vi "celcius_to_farenheit.vi"() -> ()   [LabVIEW 2019]
panel:
  in  "celcius_slide":dbl(slide) scale=0.0..100.0
  in  "?":bool
  in  "celcius":dbl
  out "Farenheat":dbl
  # "CELSIUS TO FAREINHEAT"
  # "="
  # "(or)"
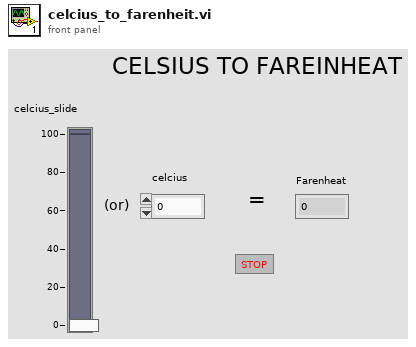
[diagram p1: front panel]
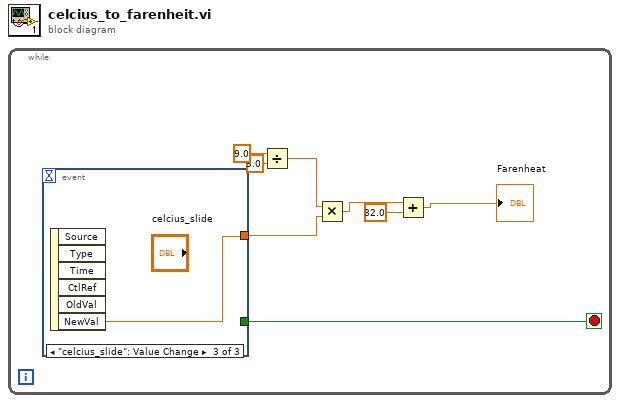
[diagram p0: block diagram]
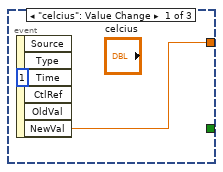
[diagram p2: hidden frame]
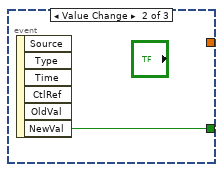
[diagram p3: hidden frame]
diagram:
  n1 = while {
    stop <- w1 stop-if-true
    n2 = event shown="[2] \"celcius_slide\": Value Change" {
      selector: _ -> [_ _ _]
      dyn-events: _ -> [_ _ _]
      timeout: _ -> [_ _ _]
      tunnel: [w9 _ w11] -> w2
      tunnel: [_ w10 _] -> w1
      event "celcius": Value Change {
        (unwired) u32 1 ("Time")
        n3 = event-data() -> ("NewVal"=w9:dbl)  [unwired: 1 in, 5 out]
      }
      event Value Change {
        n4 = event-data() -> ("NewVal"=w10:bool)  [unwired: 1 in, 5 out]
      }
      event "celcius_slide": Value Change {
        n5 = event-data() -> ("NewVal"=w11:dbl)  [unwired: 1 in, 5 out]
      }
    }
    n6 = Divide(x=9.0, y=5.0) -> (x/y=w6:dbl)
    n7 = Multiply(x=w6, y=w2) -> (x*y=w5:dbl)
    n8 = Add(x=w5, y=32.0) -> (x+y=→"Farenheat":dbl)
  }
